vi "GetMeasurements.vi"() -> ()   [LabVIEW 2016]
uses:
  <vilib>/Utility/file.llb/Write Delimited Spreadsheet (DBL).vi
panel:
  in  "DVM GIPB Address":string="7"
  out "# of Runs":i32
  in  "No B Field?":bool
  out "Remove Field":bool
  out "# of Runs":i32
  in  "+B Field Added?":bool
  out "Ready To Change Field":bool
  out "# of Runs":i32
  in  "-B Field Added?":bool
  out "Ready To Change Field":bool
  in  "DVM resource name":refnum<visa-resource-name>="Keithley2128A"
  out "?":dbl=134.169
  out "Complete?":bool
  in  "Set Current (nA)":dbl=20000.0 format="%.3f"
  in  "Voltage Measurement Path?":path=path "C:/Users/labuser/Desktop/KO Summer Research 19/Test/KO____.txt"
  in  "Current Source GPIB Address":string="12"
  # "SetUp DVM"
  # "minutes"
  # "1:"
  # "3:"
  # "2:"
  # "SetUp Current Source"
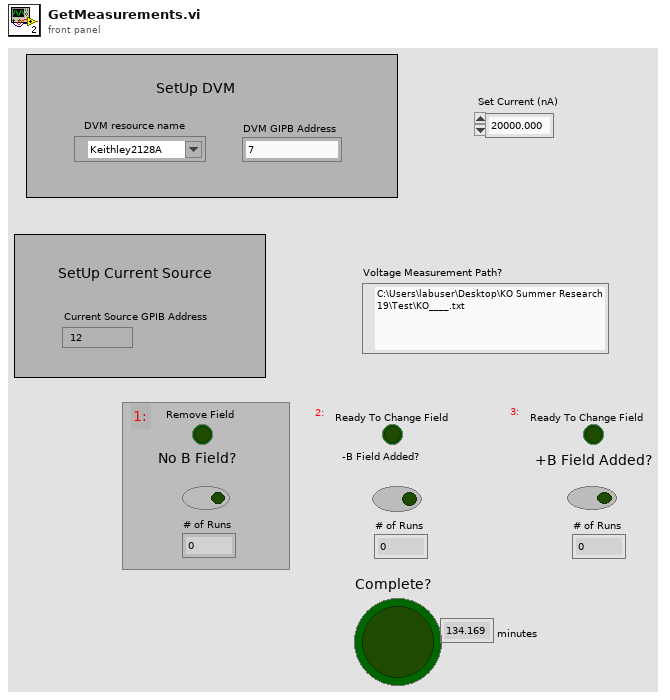
[diagram p1: front panel]
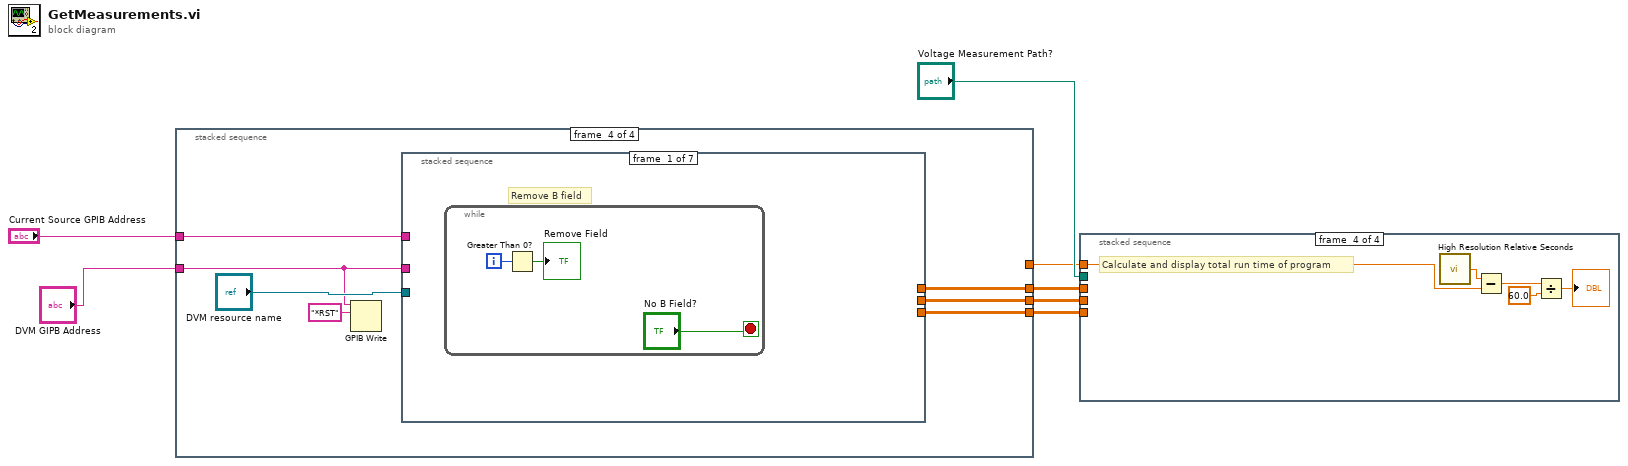
[diagram p0: block diagram]
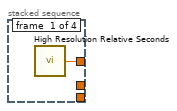
[diagram p2: hidden frame]
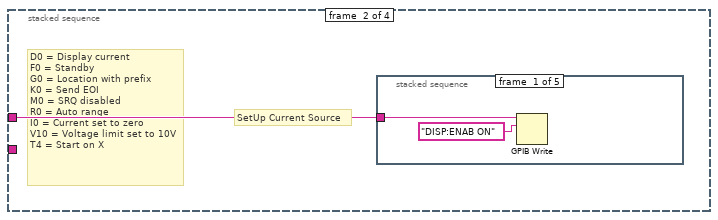
[diagram p3: hidden frame]
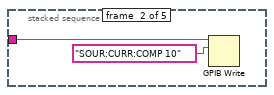
[diagram p4: hidden frame]
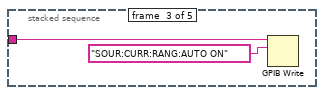
[diagram p5: hidden frame]
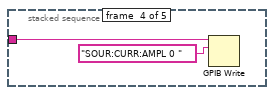
[diagram p6: hidden frame]
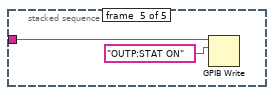
[diagram p7: hidden frame]
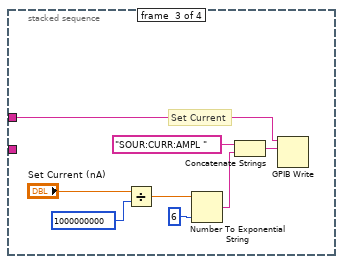
[diagram p8: hidden frame]
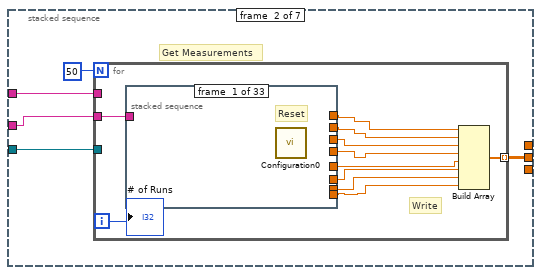
[diagram p9: hidden frame]
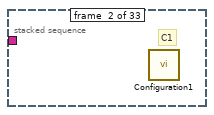
[diagram p10: hidden frame]
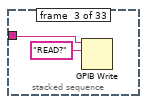
[diagram p11: hidden frame]
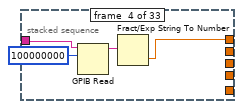
[diagram p12: hidden frame]
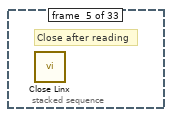
[diagram p13: hidden frame]
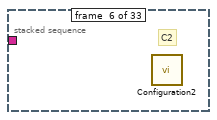
[diagram p14: hidden frame]
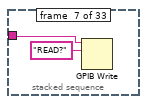
[diagram p15: hidden frame]
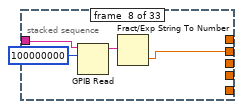
[diagram p16: hidden frame]
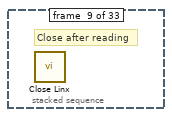
[diagram p17: hidden frame]
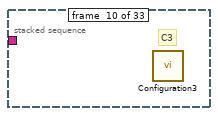
[diagram p18: hidden frame]
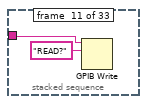
[diagram p19: hidden frame]
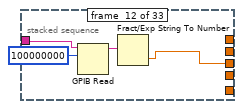
[diagram p20: hidden frame]
diagram:
  n1 = stacked-sequence {
    tunnel: "Current Source GPIB Address" -> [_ w9 w21 w34]
    tunnel: [w8 _ _ _] -> w5
    tunnel: [_ _ _ w33] -> w4
    tunnel: [_ _ _ w32] -> w3
    tunnel: [_ _ _ w31] -> w2
    tunnel: "DVM GIPB Address" -> [_ _ _ w28]
    frame #0 {
      n2 = call <vilib>:"High Resolution Relative Seconds.vi"() -> ("relative seconds"=w8:dbl)
    }
    frame #1 {
      # "SetUp Current Source"
      # "D0 = Display current\nF0 = Standby\nG0 = Location with prefix\nK0 = Send EOI\nM0 = SRQ disabled\nR0 = Auto range\nI0 = Current set to zero\nV10 = Voltage limit set to 10V\nT4 = Start on X"
      n3 = stacked-sequence {
        tunnel: w9 -> [w10 w12 w14 w16 w18]
        frame #0 {
          n4 = GPIB Write(0:w10, 1:"DISP:ENAB ON") -> ()  [unwired: 3 in, 2 out]
        }
        frame #1 {
          n5 = GPIB Write(0:w12, 1:"SOUR:CURR:COMP 10") -> ()  [unwired: 3 in, 2 out]
        }
        frame #2 {
          n6 = GPIB Write(0:w14, 1:"SOUR:CURR:RANG:AUTO ON") -> ()  [unwired: 3 in, 2 out]
        }
        frame #3 {
          n7 = GPIB Write(0:w16, 1:"SOUR:CURR:AMPL 0 ") -> ()  [unwired: 3 in, 2 out]
        }
        frame #4 {
          n8 = GPIB Write(0:w18, 1:"OUTP:STAT ON") -> ()  [unwired: 3 in, 2 out]
        }
      }
    }
    frame #2 {
      # "Set Current"
      n9 = Divide(x="Set Current (nA)", y=1000000000) -> (x/y=w23:dbl)
      n10 = Number To Exponential String(number=w23, precision (6)=6) -> (E-format string=w24:string)  [unwired: 2 in]
      n11 = Concatenate Strings("SOUR:CURR:AMPL ", w24) -> (w26:string)
      n12 = GPIB Write(0:w21, 1:w26) -> ()  [unwired: 3 in, 2 out]
    }
    frame #3 {
      n13 = GPIB Write(0:w28, 1:"*RST" ("data")) -> ()  [unwired: 3 in, 2 out]
      n14 = stacked-sequence {
        tunnel: w34 -> [_ w41 _ _ _ _ _]
        tunnel: [_ w40 _ _ _ _ _] -> w33
        tunnel: [_ _ _ w107 _ _ _] -> w32
        tunnel: [_ _ _ _ _ w147 _] -> w31
        tunnel: "DVM resource name" -> [_ w39 _ w106 _ w145 _]
        tunnel: w28 -> [_ w38 _ w105 _ w144 _]
        frame #0 {
          # "Remove B field"
          n15 = while {
            i -> [w35]
            stop <- "No B Field?" stop-if-true
            n16 = Greater Than 0?(x=w35) -> (x > 0?=→"Remove Field":bool)
          }
        }
        frame #1 {
          # "Get Measurements"
          n17 = for {
            N: 50 -> [_]
            tunnel: [w53] -> w40 mode=indexing
            tunnel: w41 -> [_]
            tunnel: w39 -> [_]
            tunnel: w38 -> [w43]
            i -> [w52]
            # "Write"
            n18 = stacked-sequence {
              tunnel: [_ _ _ w58 _ _ _ _ _ _ _ _ _ _ _ _ _ _ _ _ _ _ _ _ _ _ _ _ _ _ _ _ _] -> w51
              tunnel: [_ _ _ _ _ _ _ w63 _ _ _ _ _ _ _ _ _ _ _ _ _ _ _ _ _ _ _ _ _ _ _ _ _] -> w50
              tunnel: [_ _ _ _ _ _ _ _ _ _ _ w69 _ _ _ _ _ _ _ _ _ _ _ _ _ _ _ _ _ _ _ _ _] -> w49
              tunnel: [_ _ _ _ _ _ _ _ _ _ _ _ _ _ _ w75 _ _ _ _ _ _ _ _ _ _ _ _ _ _ _ _ _] -> w48
              tunnel: [_ _ _ _ _ _ _ _ _ _ _ _ _ _ _ _ _ _ _ w81 _ _ _ _ _ _ _ _ _ _ _ _ _] -> w47
              tunnel: [_ _ _ _ _ _ _ _ _ _ _ _ _ _ _ _ _ _ _ _ _ _ _ w87 _ _ _ _ _ _ _ _ _] -> w46
              tunnel: [_ _ _ _ _ _ _ _ _ _ _ _ _ _ _ _ _ _ _ _ _ _ _ _ _ _ _ w93 _ _ _ _ _] -> w45
              tunnel: [_ _ _ _ _ _ _ _ _ _ _ _ _ _ _ _ _ _ _ _ _ _ _ _ _ _ _ _ _ _ _ w99 _] -> w44
              tunnel: w43 -> [_ _ w54 w56 _ _ w60 w62 _ _ w66 w68 _ _ w72 w74 _ _ w78 w80 _ _ w84 w86 _ _ w90 w92 _ _ w96 w98 _]
              frame #0 {
                # "Reset"
                n19 = call "Configuration0.vi"() -> ()  [unwired: 12 in]
              }
              frame #1 {
                # "C1"
                n20 = call "Configuration1.vi"() -> ()  [unwired: 12 in]
              }
              frame #2 {
                n21 = GPIB Write(0:w54, 1:"READ?" ("data")) -> ()  [unwired: 3 in, 2 out]
              }
              frame #3 {
                n22 = GPIB Read(0:w56, 1:100000000 ("byte count")) -> (5:w59:string)  [unwired: 3 in, 2 out]
                n23 = Fract/Exp String To Number(string=w59) -> (number=w58:dbl)  [unwired: 3 in, 1 out]
              }
              frame #4 {
                # "Close after reading"
                n24 = call "Close Linx.vi"() -> ()  [unwired: 12 in]
              }
              frame #5 {
                # "C2"
                n25 = call "Configuration2.vi"() -> ()  [unwired: 12 in]
              }
              frame #6 {
                n26 = GPIB Write(0:w60, 1:"READ?" ("data")) -> ()  [unwired: 3 in, 2 out]
              }
              frame #7 {
                n27 = GPIB Read(0:w62, 1:100000000 ("byte count")) -> (5:w65:string)  [unwired: 3 in, 2 out]
                n28 = Fract/Exp String To Number(string=w65) -> (number=w63:dbl)  [unwired: 3 in, 1 out]
              }
              frame #8 {
                # "Close after reading"
                n29 = call "Close Linx.vi"() -> ()  [unwired: 12 in]
              }
              frame #9 {
                # "C3"
                n30 = call "Configuration3.vi"() -> ()  [unwired: 12 in]
              }
              frame #10 {
                n31 = GPIB Write(0:w66, 1:"READ?" ("data")) -> ()  [unwired: 3 in, 2 out]
              }
              frame #11 {
                n32 = GPIB Read(0:w68, 1:100000000 ("byte count")) -> (5:w71:string)  [unwired: 3 in, 2 out]
                n33 = Fract/Exp String To Number(string=w71) -> (number=w69:dbl)  [unwired: 3 in, 1 out]
              }
              frame #12 {
                # "Close after reading"
                n34 = call "Close Linx.vi"() -> ()  [unwired: 12 in]
              }
              frame #13 {
                # "C4"
                n35 = call "Configuration4.vi"() -> ()  [unwired: 12 in]
              }
              frame #14 {
                n36 = GPIB Write(0:w72, 1:"READ?" ("data")) -> ()  [unwired: 3 in, 2 out]
              }
              frame #15 {
                n37 = GPIB Read(0:w74, 1:100000000 ("byte count")) -> (5:w77:string)  [unwired: 3 in, 2 out]
                n38 = Fract/Exp String To Number(string=w77) -> (number=w75:dbl)  [unwired: 3 in, 1 out]
              }
              frame #16 {
                # "Close after reading"
                n39 = call "Close Linx.vi"() -> ()  [unwired: 12 in]
              }
              frame #17 {
                # "C5"
                n40 = call "Configuration5.vi"() -> ()  [unwired: 12 in]
              }
              frame #18 {
                n41 = GPIB Write(0:w78, 1:"READ?" ("data")) -> ()  [unwired: 3 in, 2 out]
              }
              frame #19 {
                n42 = GPIB Read(0:w80, 1:100000000 ("byte count")) -> (5:w83:string)  [unwired: 3 in, 2 out]
                n43 = Fract/Exp String To Number(string=w83) -> (number=w81:dbl)  [unwired: 3 in, 1 out]
              }
              frame #20 {
                # "Close after reading"
                n44 = call "Close Linx.vi"() -> ()  [unwired: 12 in]
              }
              frame #21 {
                # "C6"
                n45 = call "Configuration6.vi"() -> ()  [unwired: 12 in]
              }
              frame #22 {
                n46 = GPIB Write(0:w84, 1:"READ?" ("data")) -> ()  [unwired: 3 in, 2 out]
              }
              frame #23 {
                n47 = GPIB Read(0:w86, 1:100000000 ("byte count")) -> (5:w89:string)  [unwired: 3 in, 2 out]
                n48 = Fract/Exp String To Number(string=w89) -> (number=w87:dbl)  [unwired: 3 in, 1 out]
              }
              frame #24 {
                # "Close after reading"
                n49 = call "Close Linx.vi"() -> ()  [unwired: 12 in]
              }
              frame #25 {
                # "C7"
                n50 = call "Configuration7.vi"() -> ()  [unwired: 12 in]
              }
              frame #26 {
                n51 = GPIB Write(0:w90, 1:"READ?" ("data")) -> ()  [unwired: 3 in, 2 out]
              }
              frame #27 {
                n52 = GPIB Read(0:w92, 1:100000000 ("byte count")) -> (5:w95:string)  [unwired: 3 in, 2 out]
                n53 = Fract/Exp String To Number(string=w95) -> (number=w93:dbl)  [unwired: 3 in, 1 out]
              }
              frame #28 {
                # "Close after reading"
                n54 = call "Close Linx.vi"() -> ()  [unwired: 12 in]
              }
              frame #29 {
                # "C8"
                n55 = call "Configuration8.vi"() -> ()  [unwired: 12 in]
              }
              frame #30 {
                n56 = GPIB Write(0:w96, 1:"READ?" ("data")) -> ()  [unwired: 3 in, 2 out]
              }
              frame #31 {
                n57 = GPIB Read(0:w98, 1:100000000 ("byte count")) -> (5:w101:string)  [unwired: 3 in, 2 out]
                n58 = Fract/Exp String To Number(string=w101) -> (number=w99:dbl)  [unwired: 3 in, 1 out]
              }
              frame #32 {
                # "Close after reading"
                n59 = call "Close Linx.vi"() -> ()  [unwired: 12 in]
              }
            }
            n60 = Build Array(w51, w50, w49, w48, w47, w46, w45, w44) -> (w53:dbl[])
            "# of Runs" <- w52
          }
        }
        frame #2 {
          n61 = while {
            i -> [w103]
            stop <- "-B Field Added?" stop-if-true
            # "Add -B field"
            n62 = Greater Than 0?(x=w103) -> (x > 0?=→"Ready To Change Field":bool)
          }
        }
        frame #3 {
          n63 = for {
            N: 50 -> [_]
            tunnel: w106 -> [w115]
            tunnel: [w116] -> w107 mode=indexing
            tunnel: w105 -> [w109]
            i -> [w110]
            n64 = stacked-sequence {
              tunnel: w115 -> [_ _ _ _ _ _ _ _ _ _ _ _ _ _ _ _ _]
              tunnel: [_ _ _ w121 _ _ _ _ _ _ _ _ _ _ _ _ _] -> w114
              tunnel: [_ _ _ _ _ _ _ w126 _ _ _ _ _ _ _ _ _] -> w113
              tunnel: [_ _ _ _ _ _ _ _ _ _ _ w131 _ _ _ _ _] -> w112
              tunnel: [_ _ _ _ _ _ _ _ _ _ _ _ _ _ _ w137 _] -> w111
              tunnel: w109 -> [_ _ w118 w119 _ _ w124 w125 _ _ w130 w132 _ _ w136 w138 _]
              frame #0 {
                # "Reset"
                n65 = call "Configuration0.vi"() -> ()  [unwired: 12 in]
              }
              frame #1 {
                # "C9"
                n66 = call "Configuration9.vi"() -> ()  [unwired: 12 in]
              }
              frame #2 {
                n67 = GPIB Write(0:w118, 1:"READ?" ("data")) -> ()  [unwired: 3 in, 2 out]
              }
              frame #3 {
                n68 = GPIB Read(0:w119, 1:100000000 ("byte count")) -> (5:w122:string)  [unwired: 3 in, 2 out]
                n69 = Fract/Exp String To Number(string=w122) -> (number=w121:dbl)  [unwired: 3 in, 1 out]
              }
              frame #4 {
                # "Close after reading"
                n70 = call "Close Linx.vi"() -> ()  [unwired: 12 in]
              }
              frame #5 {
                # "C10"
                n71 = call "Configuration10.vi"() -> ()  [unwired: 12 in]
              }
              frame #6 {
                n72 = GPIB Write(0:w124, 1:"READ?" ("data")) -> ()  [unwired: 3 in, 2 out]
              }
              frame #7 {
                n73 = GPIB Read(0:w125, 1:100000000 ("byte count")) -> (5:w128:string)  [unwired: 3 in, 2 out]
                n74 = Fract/Exp String To Number(string=w128) -> (number=w126:dbl)  [unwired: 3 in, 1 out]
              }
              frame #8 {
                # "Close after reading"
                n75 = call "Close Linx.vi"() -> ()  [unwired: 12 in]
              }
              frame #9 {
                # "C11"
                n76 = call "Configuration11.vi"() -> ()  [unwired: 12 in]
              }
              frame #10 {
                n77 = GPIB Write(0:w130, 1:"READ?" ("data")) -> ()  [unwired: 3 in, 2 out]
              }
              frame #11 {
                n78 = GPIB Read(0:w132, 1:100000000 ("byte count")) -> (5:w134:string)  [unwired: 3 in, 2 out]
                n79 = Fract/Exp String To Number(string=w134) -> (number=w131:dbl)  [unwired: 3 in, 1 out]
              }
              frame #12 {
                # "Close after reading"
                n80 = call "Close Linx.vi"() -> ()  [unwired: 12 in]
              }
              frame #13 {
                # "C12"
                n81 = call "Configuration12.vi"() -> ()  [unwired: 12 in]
              }
              frame #14 {
                n82 = GPIB Write(0:w136, 1:"READ?" ("data")) -> ()  [unwired: 3 in, 2 out]
              }
              frame #15 {
                n83 = GPIB Read(0:w138, 1:100000000 ("byte count")) -> (5:w140:string)  [unwired: 3 in, 2 out]
                n84 = Fract/Exp String To Number(string=w140) -> (number=w137:dbl)  [unwired: 3 in, 1 out]
              }
              frame #16 {
                # "Close after reading"
                n85 = call "Close Linx.vi"() -> ()  [unwired: 12 in]
              }
            }
            n86 = Build Array(w114, w113, w112, w111) -> (w116:dbl[])
            "# of Runs" <- w110
          }
        }
        frame #4 {
          # "Change to +B Field"
          n87 = while {
            i -> [w141]
            stop <- "+B Field Added?" stop-if-true
            n88 = Greater Than 0?(x=w141) -> (x > 0?=→"Ready To Change Field":bool)
          }
        }
        frame #5 {
          n89 = for {
            N: 50 -> [_]
            tunnel: w145 -> [_]
            tunnel: [w154] -> w147 mode=indexing
            tunnel: w144 -> [w148]
            i -> [w153]
            n90 = stacked-sequence {
              tunnel: [_ _ _ w159 _ _ _ _ _ _ _ _ _ _ _ _ _] -> w152
              tunnel: [_ _ _ _ _ _ _ w164 _ _ _ _ _ _ _ _ _] -> w151
              tunnel: [_ _ _ _ _ _ _ _ _ _ _ _ _ _ _ w176 _] -> w149
              tunnel: [_ _ _ _ _ _ _ _ _ _ _ w170 _ _ _ _ _] -> w150
              tunnel: w148 -> [_ _ w155 w157 _ _ w161 w163 _ _ w167 w169 _ _ w173 w175 _]
              frame #0 {
                # "Reset"
                n91 = call "Configuration0.vi"() -> ()  [unwired: 12 in]
              }
              frame #1 {
                # "C13"
                n92 = call "Configuration9.vi"() -> ()  [unwired: 12 in]
              }
              frame #2 {
                n93 = GPIB Write(0:w155, 1:"READ?" ("data")) -> ()  [unwired: 3 in, 2 out]
              }
              frame #3 {
                n94 = GPIB Read(0:w157, 1:100000000 ("byte count")) -> (5:w160:string)  [unwired: 3 in, 2 out]
                n95 = Fract/Exp String To Number(string=w160) -> (number=w159:dbl)  [unwired: 3 in, 1 out]
              }
              frame #4 {
                # "Close after reading"
                n96 = call "Close Linx.vi"() -> ()  [unwired: 12 in]
              }
              frame #5 {
                # "C14"
                n97 = call "Configuration10.vi"() -> ()  [unwired: 12 in]
              }
              frame #6 {
                n98 = GPIB Write(0:w161, 1:"READ?" ("data")) -> ()  [unwired: 3 in, 2 out]
              }
              frame #7 {
                n99 = GPIB Read(0:w163, 1:100000000 ("byte count")) -> (5:w166:string)  [unwired: 3 in, 2 out]
                n100 = Fract/Exp String To Number(string=w166) -> (number=w164:dbl)  [unwired: 3 in, 1 out]
              }
              frame #8 {
                # "Close after reading"
                n101 = call "Close Linx.vi"() -> ()  [unwired: 12 in]
              }
              frame #9 {
                # "C15"
                n102 = call "Configuration11.vi"() -> ()  [unwired: 12 in]
              }
              frame #10 {
                n103 = GPIB Write(0:w167, 1:"READ?" ("data")) -> ()  [unwired: 3 in, 2 out]
              }
              frame #11 {
                n104 = GPIB Read(0:w169, 1:100000000 ("byte count")) -> (5:w172:string)  [unwired: 3 in, 2 out]
                n105 = Fract/Exp String To Number(string=w172) -> (number=w170:dbl)  [unwired: 3 in, 1 out]
              }
              frame #12 {
                # "Close after reading"
                n106 = call "Close Linx.vi"() -> ()  [unwired: 12 in]
              }
              frame #13 {
                # "C16"
                n107 = call "Configuration12.vi"() -> ()  [unwired: 12 in]
              }
              frame #14 {
                n108 = GPIB Write(0:w173, 1:"READ?" ("data")) -> ()  [unwired: 3 in, 2 out]
              }
              frame #15 {
                n109 = GPIB Read(0:w175, 1:100000000 ("byte count")) -> (5:w178:string)  [unwired: 3 in, 2 out]
                n110 = Fract/Exp String To Number(string=w178) -> (number=w176:dbl)  [unwired: 3 in, 1 out]
              }
              frame #16 {
                # "Close after reading"
                n111 = call "Close Linx.vi"() -> ()  [unwired: 12 in]
              }
            }
            n112 = Build Array(w152, w151, w150, w149) -> (w154:dbl[])
            "# of Runs" <- w153
          }
        }
        frame #6 {
          "Complete?" <- TRUE
        }
      }
    }
  }
  n113 = stacked-sequence {
    tunnel: "Voltage Measurement Path?" -> [w181 w187 w193 _]
    tunnel: w4 -> [w180 _ _ _]
    tunnel: w3 -> [_ w186 _ _]
    tunnel: w5 -> [_ _ _ w198]
    tunnel: w2 -> [_ _ w192 _]
    frame #0 {
      # "Write voltages (V) to file (.txt)"
      n114 = call-poly <vilib>:"Write Delimited Spreadsheet.vi"("file path (dialog if empty)"=w181, "format (%.3f)"="%16.14f", "2D data"=w180, "append to file? (new file:F)"=TRUE ("append to file? (F)"), "transpose? (no:F)"=FALSE ("transpose? (F)"), "delimiter (\\t)"="," ("delimiter (\\t)")) -> ()  [unwired: 8 in, 2 out]
    }
    frame #1 {
      # "Write voltages (V) to file (.txt)"
      n115 = call-poly <vilib>:"Write Delimited Spreadsheet.vi"("file path (dialog if empty)"=w187, "format (%.3f)"="%16.14f", "2D data"=w186, "append to file? (new file:F)"=TRUE ("append to file? (F)"), "transpose? (no:F)"=FALSE ("transpose? (F)"), "delimiter (\\t)"="," ("delimiter (\\t)")) -> ()  [unwired: 8 in, 2 out]
    }
    frame #2 {
      n116 = call-poly <vilib>:"Write Delimited Spreadsheet.vi"("file path (dialog if empty)"=w193, "format (%.3f)"="%16.14f", "2D data"=w192, "append to file? (new file:F)"=TRUE ("append to file? (F)"), "transpose? (no:F)"=FALSE ("transpose? (F)"), "delimiter (\\t)"="," ("delimiter (\\t)")) -> ()  [unwired: 8 in, 2 out]
    }
    frame #3 {
      # "Calculate and display total run time of program"
      n117 = call <vilib>:"High Resolution Relative Seconds.vi"() -> ("relative seconds"=w202:dbl)
      n118 = Subtract(x=w202, y=w198) -> (x-y=w201:dbl)
      n119 = Divide(x=w201, y=60.0) -> (x/y=→"?":dbl)
    }
  }
